vi "ADC - Enable Analog Input Channel.vi"(8 "error in (no error)":errorcluster, 10 "Analog Input Channel Number":i32, 11 "TCP Network Connection in":refnum<k5>) -> (0 "error out":errorcluster, 3 "TCP Network Connection out":refnum<k5>)   [LabVIEW 2020]
doc: "Send a TCP command to the DAQ which enables an analog input channel."
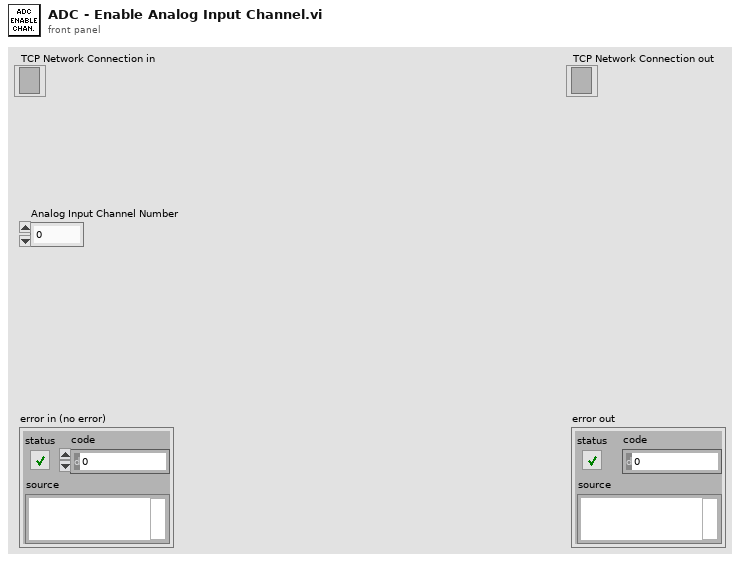
[diagram p1: front panel]
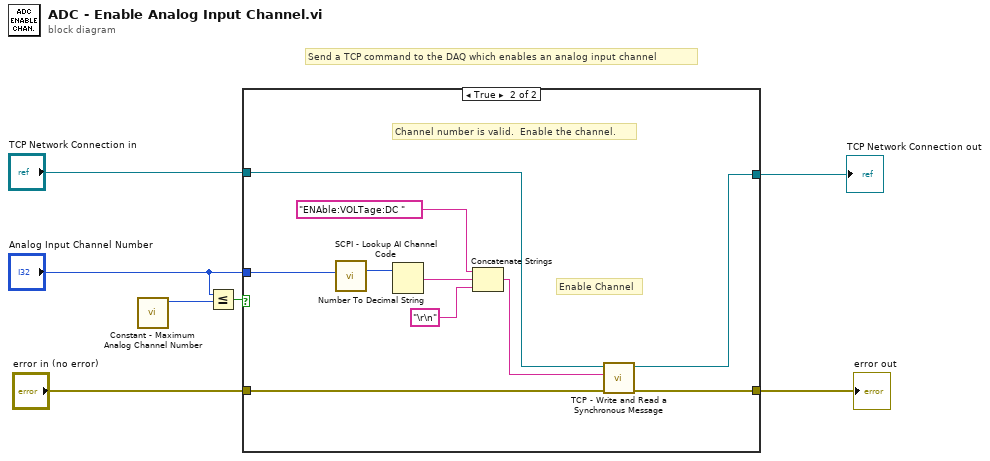
[diagram p0: block diagram]
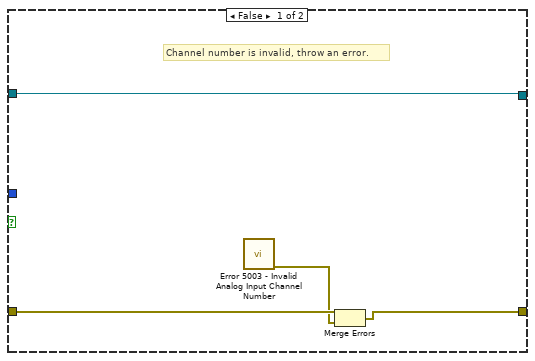
[diagram p2: hidden frame]
diagram:
  # "Send a TCP command to the DAQ which enables an analog input channel"
  n1 = call "Constant - Maximum Analog Channel Number.vi"() -> ("Maximum Channel"=w2:i32)  [unwired: 11 in]
  n2 = Less Or Equal?(x="Analog Input Channel Number", y=w2) -> (x <= y?=w1:bool)
  n3 = case shown="True" w1 {
    tunnel: [w10 w21] -> w7
    tunnel: [w8 w20] -> w6
    tunnel: "error in (no error)" -> [w11 w14]
    tunnel: "TCP Network Connection in" -> [w8 w13]
    tunnel: "Analog Input Channel Number" -> [_ w12]
    frame False {
      # "Channel number is invalid, throw an error."
      n4 = call "Error 5003 - Invalid Analog Input Channel Number.vi"() -> ("error out"=w9:errorcluster)  [unwired: 11 in]
      n5 = Merge Errors(w11, w9) -> (w10:errorcluster)
    }
    frame True {
      # "Channel number is valid.  Enable the channel."
      # "Enable Channel"
      n6 = call "SCPI - Lookup AI Channel Code.vi"("Analog Input Channel Number"=w12) -> ("Channel Code"=w15:i32)  [unwired: 10 in]
      n7 = Number To Decimal String(number=w15) -> (decimal integer string=w17:string)  [unwired: 1 in]
      n8 = Concatenate Strings("ENAble:VOLTage:DC " ("Message to Send"), w17, "\r\n" ("string")) -> (w19:string)
      n9 = call "TCP - Write and Read a Synchronous Message.vi"("error in"=w14, "Message to Send"=w19, "TCP Network Connection in"=w13) -> ("error out"=w21:errorcluster, "TCP Network Connection out"=w20:refnum<k5>)  [unwired: 6 in, 1 out]
    }
  }
  "error out" <- w7
  "TCP Network Connection out" <- w6
